vi "WPI_Custom_CameraSend Images To PC Loop.vi"(8 "error in (no error)":errorcluster, 9 "CameraDevRef 2":T1, 11 "CameraDevRef":T1) -> ()   [LabVIEW 2015]
doc: "This VI is used to send images to the dashboard using the second enet port on the 8 slot controller. This is provided for compatibility, but is higher overhead than using the Camera MJPG approach.\n\nThis software is licensed. Open the labview\\readme\\WPI Robotics Library Open Source License.txt file for more information."
uses:
  <vilib>/Rock Robotics/WPI/Camera/WPI_CameraDevRef.ctl
  <vilib>/Rock Robotics/SystemInterfaces/NetworkCommunication/NetComm_UsageReport_ResourceType.ctl
  Robot Global Data.vi
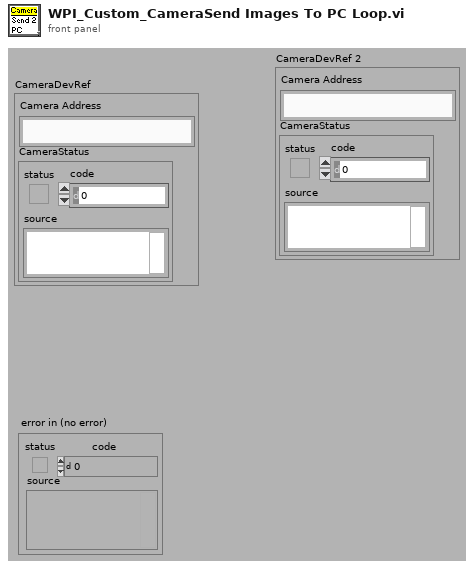
[diagram p1: front panel]
types:
  T1 = typedef "WPI_CameraDevRef.ctl" = cluster{"Camera Address":string, "CameraStatus":errorcluster}
  T2 = cluster{"fps":i32, "compression":i32, "compression 2":i32}
  T3 = typedef "NetComm_UsageReport_ResourceType.ctl" = enum8{"Controller", "Module", "Language", "CANPlugin", "Accelerometer", "ADXL345", "AnalogChannel", "AnalogTrigger", "AnalogTriggerOutput", "CANJaguar", "Compressor", "Counter", "Dashboard", "DigitalInput", "DigitalOutput", "DriverStationCIO", "DriverStationEIO", "DriverStationLCD", "Encoder", "GearTooth", "Gyro", "I2C", "Framework", "Jaguar", "Joystick", "Kinect", "KinectStick", "PIDController", "Preferences", "PWM", "Relay", "RobotDrive", "SerialPort", "Servo", "Solenoid", "SPI", "Task", "Ultrasonic", "Victor", "Button", "Command", "AxisCamera", "PCVideoServer", "SmartDashboard", "Talon", "HiTechnicColorSensor", "HiTechnicAccel", "HiTechnicCompass", "SRF08", "AnalogOutput", "Victor SP", "Talon SRX", "CAN Talon SRX", "ADXL362 Accel", "ADXRS450 Gyro", "Rev SPARK", "Mindsensors SD540", "Digital Filter"}
  T4 = enum16{"Update Mode", "Get Image", "Get Image Data"}
  T5 = typedef "Image Type" = u32
  T6 = typedef "IMAQ Image.ctl" = refnum<image>
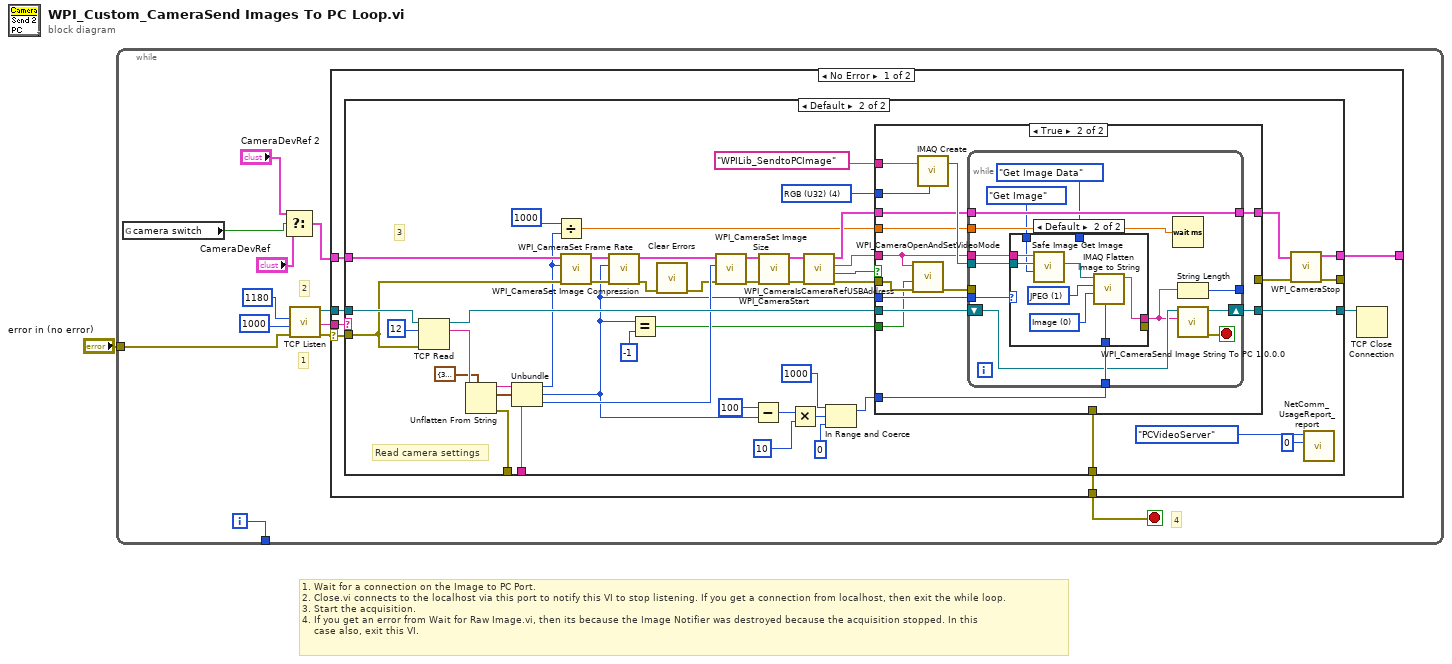
[diagram p0: block diagram]
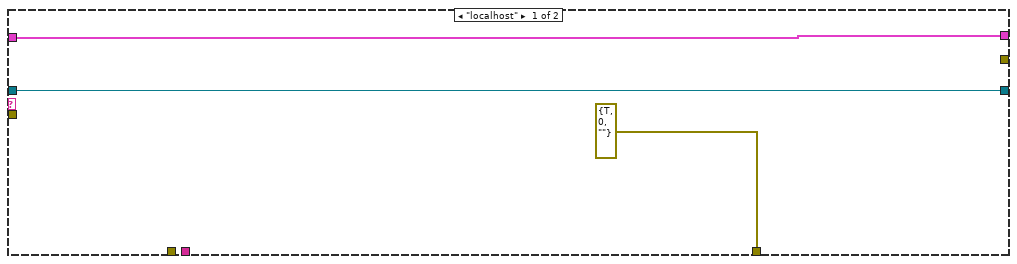
[diagram p2: hidden frame]
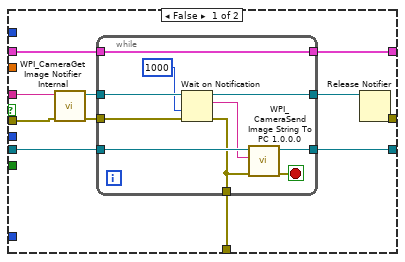
[diagram p3: hidden frame]
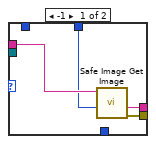
[diagram p4: hidden frame]
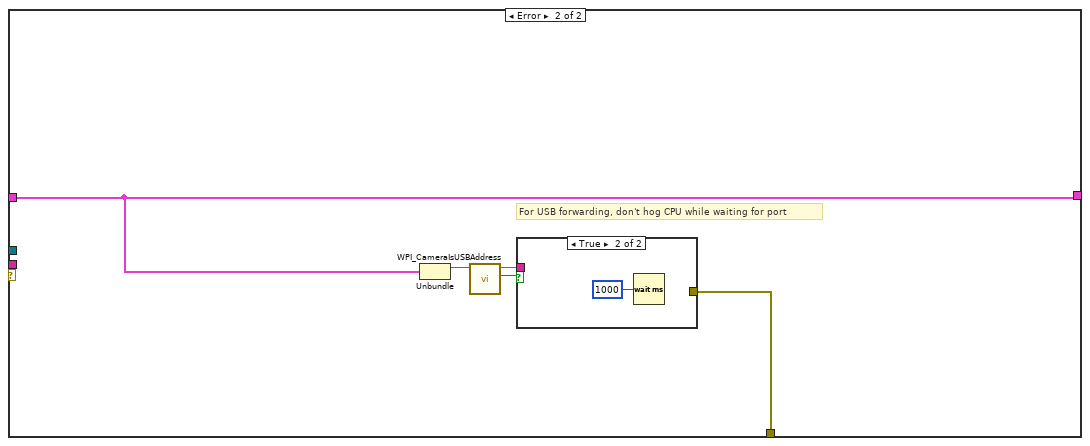
[diagram p5: hidden frame]
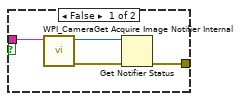
[diagram p6: hidden frame]
diagram:
  # "1. Wait for a connection on the Image to PC Port.\n2. Close.vi connects to the localhost via this port to notify this VI to stop listening. If you get a connection from localhost, then exit the while loop.\n3. Start the acquisition.\n4. If you get an error from Wait for Raw Image.vi, then its because the Image Notifier was destroyed because the acquisition stopped. In this\n    case also, exit this VI."
  n1 = while {
    tunnel: "error in (no error)" -> [w12]
    tunnel: [w6] -> _
    i -> [w6]
    stop <- w10 stop-if-true
    # "4"
    # "1"
    # "2"
    n2 = global read "Robot Global Data.vi" "camera switch"() -> (w2:bool)
    n3 = Select(t="CameraDevRef 2", s=w2, f="CameraDevRef") -> (s? t:f=w5:T1)
    n4 = call <vilib>:"TCP Listen.vi"("error in (no error)"=w12, "timeout ms (wait forever: -1)"=u16 1000 ("port"), "port"=u16 1180) -> ("error out"=w8:errorcluster, "remote address"=w13:string, "connection ID"=w11:refnum<k5>)  [unwired: 1 in, 5 out]
    n5 = case shown="No Error" w8 {
      selector: w8 -> [w14 _]
      tunnel: [w20 w134] -> _
      tunnel: w13 -> [w19 _]
      tunnel: w5 -> [w18 w134]
      tunnel: w11 -> [w17 _]
      tunnel: [w16 w135] -> w10
      frame No Error {
        n6 = case shown="Default" w19 {
          tunnel: [w23 w68] -> w20
          tunnel: w18 -> [w23 w50]
          tunnel: w14 -> [_ w46]
          tunnel: w17 -> [w21 w54]
          tunnel: [errorcluster {"status"=TRUE, "code"=0, "source"=""} ("error out 2") w70] -> w16
          tunnel: [w21 w69] -> w15
          tunnel: [_ w67] -> _
          tunnel: [_ w25] -> _
          tunnel: [_ w24] -> _
          frame "localhost" {
          }
          frame Default {
            w61 = T5 4 items=["Grayscale (U8)", "Grayscale (I16)", "Grayscale (SGL)", "Complex (CSG)", "RGB (U32)", "HSL (U32)", "RGB (U64)", "Grayscale (U16)"] ("Image Type")
            # "Read camera settings"
            # "3"
            n7 = TCP Read(connection ID=w54, bytes to read=12, error in (no error)=w46) -> (connection ID out=w53:refnum<k5>, data out=w51:string)  [unwired: 2 in, 1 out]
            n8 = Unflatten From String(type=T2 {"fps"=30, "compression"=32, "compression 2"=32} ("Camera Settings"), binary string=w51) -> (rest of the binary string=w24:string, value=w43:T2, error out=w25:errorcluster)  [unwired: 3 in]
            n9 = Unbundle(w43) -> ("fps"=w40:i32, "compression"=w29:i32, "compression 2"=w42:i32)
            n10 = Divide(x=u16 1000 ("port"), y=w40) -> (x/y=w39:dbl)
            n11 = call <vilib>:"WPI_CameraSet Frame Rate.vi"("error in (no error)"=w46, "Frame Rate (fps)"=w40, "CameraDevRef"=w50) -> ("error out"=w45:errorcluster, "CameraDevRef Out"=w49:T1)  [unwired: 7 in]
            n12 = call <vilib>:"WPI_CameraSet Image Compression.vi"("error in (no error)"=w45, "Compression"=w29, "CameraDevRef"=w49) -> ("error out"=w27:errorcluster, "CameraDevRef Out"=w48:T1)  [unwired: 7 in]
            n13 = Equal?(x=w29, y=-1) -> (x = y?=w28:bool)
            n14 = call <vilib>:"Clear Errors.vi"("error in (no error)"=w27) -> ("error out"=w26:errorcluster)  [unwired: 5 in, 1 out]
            n15 = call <vilib>:"WPI_CameraSet Image Size.vi"("error in (no error)"=w26, "Image Size"=w42, "CameraDevRef"=w48) -> ("error out"=w44:errorcluster, "CameraDevRef Out"=w47:T1)  [unwired: 7 in]
            n16 = Subtract(x=100, y=w29) -> (x-y=w34:i32)
            n17 = call <vilib>:"WPI_CameraStart.vi"("error in (no error)"=w44, "CameraDevRef"=w47) -> ("error out"=w58:errorcluster, "CameraDevRef"=w56:T1)  [unwired: 8 out]
            n18 = Multiply(x=w34, y=10) -> (x*y=w36:i32)
            n19 = call <vilib>:"WPI_CameraIsCameraRefUSBAddress.vi"("error in (no error)"=w58, "CameraDevRef"=w56) -> ("error out"=w57:errorcluster, "USB?"=w59:bool, "Camera Address Out"=w60:string, "CameraDevRef out"=w55:T1)  [unwired: 6 in]
            n20 = In Range and Coerce(upper limit=1000, x=w36, lower limit=0) -> (coerced(x)=w32:i32)  [unwired: 1 out]
            n21 = case shown="True" w59 {
              tunnel: w53 -> [w81 w105]
              tunnel: [w80 _] -> w70
              tunnel: [w79 w104] -> w69
              tunnel: w57 -> [w78 w95]
              tunnel: w60 -> [w76 w94]
              tunnel: [w75 w99] -> w66
              tunnel: w55 -> [w74 w100]
              tunnel: [w72 _] -> w65
              tunnel: "WPILib_SendtoPCImage" -> [_ w102]
              tunnel: w61 -> [_ w101]
              tunnel: w32 -> [_ w98]
              tunnel: w39 -> [_ w97]
              tunnel: w29 -> [_ w96]
              tunnel: w28 -> [_ w92]
              frame False {
                n22 = call <vilib>:"WPI_CameraGet Image Notifier Internal.vi"("error in (no error)"=w78, "Camera Address"=w76) -> ("error out"=w77:errorcluster, "Image Notifier"=w73:refnum<notifier>)  [unwired: 8 out]
                n23 = while {
                  tunnel: w77 -> [w87]
                  tunnel: w81 -> [w91]
                  tunnel: [w84] -> w80
                  tunnel: [w89] -> w79
                  tunnel: [w88] -> w75
                  tunnel: w74 -> [w88]
                  tunnel: w73 -> [w86]
                  tunnel: [w82] -> w71
                  stop <- w90 stop-if-true
                  n24 = Wait on Notification(notifier=w86, timeout in ms (-1)=1000 ("Timeout in ms (-1)"), error in (no error)=w87) -> (notifier out=w82:refnum<notifier>, notification=w85:string, error out=w84:errorcluster)  [unwired: 2 out]
                  n25 = call <vilib>:"WPI_CameraSend Image String To PC 1.0.0.0.vi"("error in (no error)"=w84, "String"=w85, "TCP Connection ID"=w91) -> ("error out"=w90:errorcluster, "TCP Connection ID out"=w89:refnum<k5>)  [unwired: 7 out]
                }
                n26 = Release Notifier(notifier=w71) -> (error out=w72:errorcluster)  [unwired: 1 in, 3 out]
              }
              frame True {
                n27 = call <vilib>:"WPI_CameraOpenAndSetVideoMode.vi"("error in (no error)"=w95, "USB JPEG"=w92, "Camera Address Out"=w94) -> ("error out"=w93:errorcluster)  [unwired: 8 in]
                n28 = call "IMAQ Create"("Image Name"=w102, "Image Type"=w101) -> ("New Image"=w103:T6)  [unwired: 3 in, 1 out]
                n29 = while {
                  tunnel: w94 -> [w117]
                  shift-right: [w118] -> w104
                  shift-left: w105 -> [w111]
                  tunnel: w103 -> [w116]
                  tunnel: [w114] -> w99
                  tunnel: w100 -> [w114]
                  tunnel: w98 -> [w113]
                  tunnel: w97 -> [w112]
                  tunnel: [w109] -> _
                  tunnel: w96 -> [w108]
                  tunnel: w93 -> [_]
                  stop <- w115 stop-if-true
                  n30 = case shown="Default" w108 {
                    tunnel: [w121 w130] -> w110
                    tunnel: w117 -> [w122 w126]
                    tunnel: w116 -> [_ w125]
                    tunnel: w113 -> [_ w127]
                    tunnel: [w120 _] -> _
                    tunnel: T4."Get Image Data" ("Operation") -> [w119 _]
                    tunnel: T4."Get Image" ("Operation") -> [_ w123]
                    frame -1 {
                      n31 = call <vilib>:"Safe Image Get Image.vi"("Operation"=w119, "Session In"=w122) -> ("error out"=w120:errorcluster, "Image Data String"=w121:string)  [unwired: 6 in, 2 out]
                    }
                    frame Default {
                      w128 = 0 items=["Image", "Image and Vision Info", "Reference to Image"] ("Type of Flatten (Image and Vision Info)")
                      w129 = 1 items=["None", "JPEG", "PACKED BINARY"] ("Compression (None)")
                      n32 = call <vilib>:"Safe Image Get Image.vi"("Operation"=w123, "Image In"=w125, "Session In"=w126) -> ("Image Out"=w124:T6)  [unwired: 5 in, 3 out]
                      n33 = call "IMAQ Flatten Image to String"("Quality (750)"=w127, "Type of Flatten (Image and Vision Info)"=w128, "Compression (None)"=w129, "Image"=w124) -> ("Data String"=w130:string)  [unwired: 6 in, 1 out]
                    }
                  }
                  n34 = Wait (ms)(milliseconds to wait=w112) -> ()  [unwired: 1 out]
                  n35 = String Length(string=w110) -> (length=w109:i32)
                  n36 = call <vilib>:"WPI_CameraSend Image String To PC 1.0.0.0.vi"("String"=w110, "TCP Connection ID"=w111) -> ("error out"=w115:errorcluster, "TCP Connection ID out"=w118:refnum<k5>)  [unwired: 1 in, 7 out]
                }
              }
            }
            n37 = call <vilib>:"WPI_CameraStop.vi"("error in (no error)"=w65, "CameraDevRef"=w66) -> ("error out"=w67:errorcluster, "CameraDevRef"=w68:T1)  [unwired: 8 out]
            n38 = call <vilib>:"NetComm_UsageReport_report.vi"("Instance Number"=u8 0, "Resource Type"=NetComm_UsageReport_ResourceType."PCVideoServer") -> ()  [unwired: 10 in]
          }
        }
        n39 = TCP Close Connection(connection ID=w15) -> ()  [unwired: 1 in, 3 out]
      }
      frame Error {
        # "For USB forwarding, don't hog CPU while waiting for port"
        n40 = Unbundle(w134) -> ("Camera Address"=w133:string)  [unwired: 1 out]
        n41 = call <vilib>:"WPI_CameraIsUSBAddress.vi"("Camera Address In"=w133) -> ("USB?"=w131:bool, "Camera Address Out"=w132:string)  [unwired: 8 in, 1 out]
        n42 = case shown="True" w131 {
          tunnel: [w139 _] -> w135
          tunnel: w132 -> [w136 _]
          frame False {
            n43 = call <vilib>:"WPI_CameraGet Acquire Image Notifier Internal.vi"("Camera Address"=w136) -> ("error out"=w137:errorcluster, "Acquire Image Notifier"=w138:refnum<notifier>)  [unwired: 1 in, 8 out]
            n44 = Get Notifier Status(notifier=w138, error in (no error)=w137) -> (error out=w139:errorcluster)  [unwired: 4 out]
          }
          frame True {
            n45 = Wait (ms)(milliseconds to wait=u32 1000) -> ()  [unwired: 1 out]
          }
        }
      }
    }
  }
